vi "1TableGenerateHeaders.vi"(7 "HeaderPrefix":string, 8 "error in (no error)":errorcluster, 11 "Cluster Variant":variant) -> (0 "error out":errorcluster, 1 "LV Data Types":T1[](array[typedef]) format="%.0x", 2 "Headers":string[](array[string]), 3 "Table Name":string)   [LabVIEW 2014, in "TableLogger_Actor.lvlib" / "TableLogger_Actor.lvclass"]
uses:
  TableLogger_Actor.lvclass
  <userlib>/_OpenG.lib/lvdata/lvdata.llb/Type Descriptor Enumeration__ogtk.ctl
panel:
  # "Connector Pane"
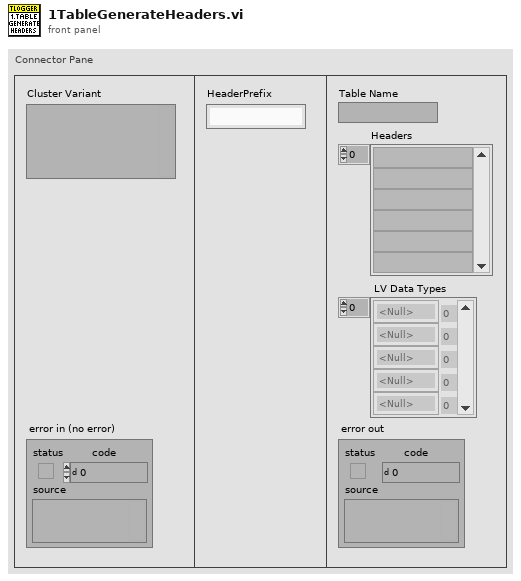
[diagram p1: front panel]
types:
  T1 = typedef "Type Descriptor Enumeration__ogtk.ctl" = enum8{"<Null>", "I8", "I16", "I32", "I64", "U8", "U16", "U32", "U64", "SGL", "DBL", "EXT", "CSG", "CDB", "CXT", "0x0F", "0x10", "0x11", "0x12", "0x13", "0x14", "Enum U8", "Enum U16", "Enum U32", "Enum U64", "SGL PQ", "DBL PQ", "EXT PQ", "CSG PQ", "CDB PQ", "CXT PQ", "0x1F", "0x20", "Boolean", "0x22", "0x23", "0x24", "0x25", "0x26", "0x27", "0x28", "0x29", "0x2A", "0x2B", "0x2C", "0x2D", "0x2E", "0x2F", "String", "0x31", "Path", "Pict", "0x34", "0x35", "0x36", "DAQ", "0x38", "0x39", "0x3A", "0x3B", "0x3C", "0x3D", "0x3E", "0x3F", "Array", "0x41", "0x42", "0x43", "0x44", "0x45", "0x46", "0x47", "0x48", "0x49", "0x4A", "0x4B", "0x4C", "0x4D", "0x4E", "0x4F", "Cluster", "0x51", "0x52", "Variant", "Waveform", "0x55", "0x56", "0x57", "0x58", "0x59", "0x5A", "0x5B", "0x5C", "0x5D", "0x5E", "0x5F", "0x60", "0x61", "0x62", "0x63", "0x64", "0x65", "0x66", "0x67", "0x68", "0x69", "0x6A", "0x6B", "0x6C", "0x6D", "0x6E", "0x6F", "Refnum"}
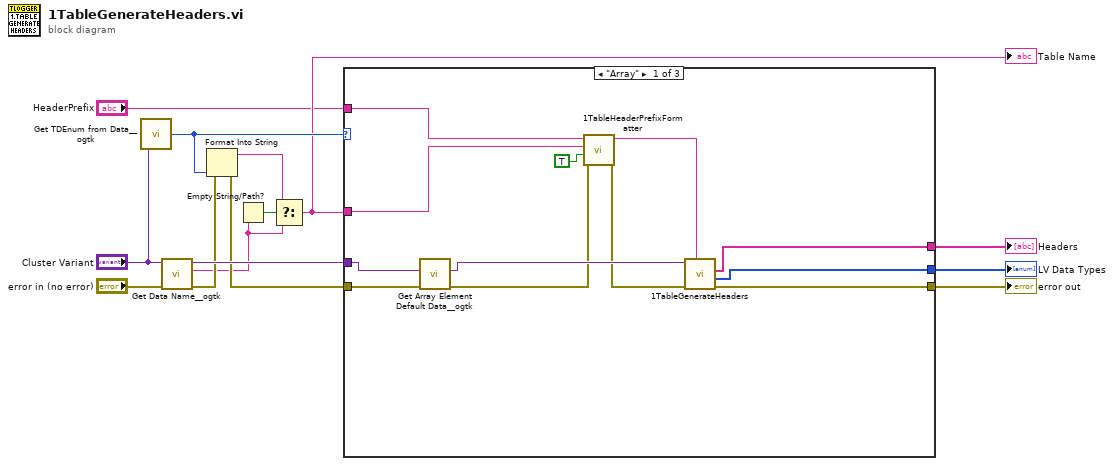
[diagram p0: block diagram]
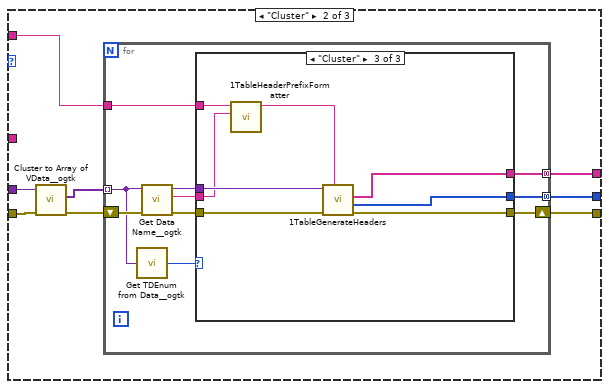
[diagram p2: hidden frame]
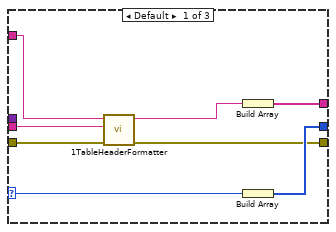
[diagram p3: hidden frame]
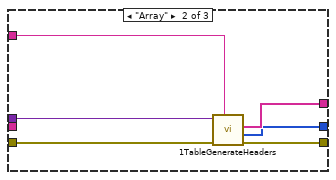
[diagram p4: hidden frame]
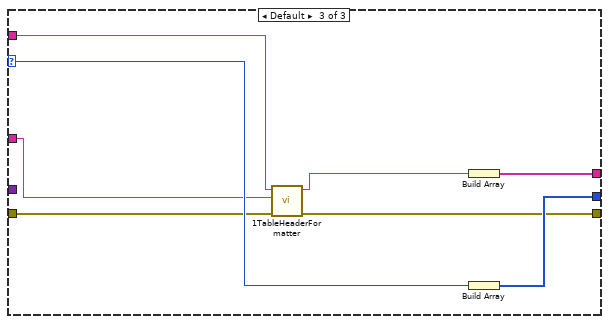
[diagram p5: hidden frame]
diagram:
  n1 = call <userlib>:"Get TDEnum from Data__ogtk.vi"("Data"="Cluster Variant") -> ("Type Descriptor Enumeration"=w7:T1)  [unwired: 4 in]
  n2 = call <userlib>:"Get Data Name__ogtk.vi"("error in (no error)"="error in (no error)", "Data"="Cluster Variant") -> ("error out"=w5:errorcluster, "Data Name"=w3:string, "Data dup"=w9:variant)  [unwired: 7 in]
  n3 = Format Into String(error in=w5, w7) -> (resulting string=w6:string, error out=w4:errorcluster)  [unwired: 2 in]
  n4 = Empty String/Path?(string/path=w3) -> (empty?=w8:bool)
  n5 = Select(t=w6, s=w8, f=w3) -> (s? t:f=w2:string)
  "Table Name" <- w2
  n6 = case shown="\"Array\"" w7 {
    selector: w7 -> [_ _ w72]
    tunnel: w9 -> [w22 w33 _]
    tunnel: [w26 w34 w74] -> w14
    tunnel: w4 -> [w23 w28 w71]
    tunnel: [w25 w30 w70] -> w13
    tunnel: [w21 w29 w73] -> w12
    tunnel: "HeaderPrefix" -> [w20 w27 w69]
    tunnel: w2 -> [w19 _ w68]
    frame "Array" {
      n7 = call <userlib>:"Get Array Element Default Data__ogtk.vi"("error in (no error)"=w23, "Array"=w22) -> ("error out"=w16:errorcluster, "Array Element Default Data"=w24:variant)  [unwired: 8 in]
      n8 = call "1TableHeaderPrefixFormatter.vi"("error in"=w16, "Array?"=TRUE, "Added HeaderPrefix"=w19, "Existing HeaderPrefix"=w20) -> ("error out"=w15:errorcluster, "HeaderPrefix"=w18:string)  [unwired: 6 in]
      n9 = call "1TableGenerateHeaders.vi"("HeaderPrefix"=w18, "error in (no error)"=w15, "Cluster Variant"=w24) -> ("error out"=w25:errorcluster, "LV Data Types"=w21:T1[], "Headers"=w26:string[])  [unwired: 5 in, 1 out]
    }
    frame "Cluster" {
      n10 = call <userlib>:"Cluster to Array of VData__ogtk.vi"("error in (no error)"=w28, "Cluster"=w33) -> ("error out"=w31:errorcluster, "Array of VData"=w32:variant[])  [unwired: 8 in]
      n11 = for {
        tunnel: w32 -> [w38] mode=indexing
        tunnel: [w44] -> w34 mode=concatenating
        shift-right: [w43] -> w30
        shift-left: w31 -> [w40]
        tunnel: [w41] -> w29 mode=concatenating
        tunnel: w27 -> [w35]
        n12 = call <userlib>:"Get TDEnum from Data__ogtk.vi"("Data"=w38) -> ("Type Descriptor Enumeration"=w42:T1)  [unwired: 4 in]
        n13 = call <userlib>:"Get Data Name__ogtk.vi"("error in (no error)"=w40, "Data"=w38) -> ("error out"=w39:errorcluster, "Data Name"=w36:string, "Data dup"=w37:variant)  [unwired: 7 in]
        n14 = case shown="\"Cluster\"" w42 {
          selector: w42 -> [w50 _ _]
          tunnel: w37 -> [_ w57 w66]
          tunnel: [w52 w58 w63] -> w44
          tunnel: w39 -> [w49 w56 w65]
          tunnel: [w48 w55 w64] -> w43
          tunnel: [w51 w54 w62] -> w41
          tunnel: w36 -> [w46 _ w60]
          tunnel: w35 -> [w47 w53 w61]
          frame Default {
            n15 = call "1TableHeaderFormatter.vi"("error in (no error)"=w49, "Data Name"=w46, "HeaderPrefix"=w47) -> ("error out"=w48:errorcluster, "HeaderOut"=w45:string)  [unwired: 7 in]
            n16 = Build Array(w45) -> (w52:string[])
            n17 = Build Array(w50) -> (w51:T1[])
          }
          frame "Array" {
            n18 = call "1TableGenerateHeaders.vi"("HeaderPrefix"=w53, "error in (no error)"=w56, "Cluster Variant"=w57) -> ("error out"=w55:errorcluster, "LV Data Types"=w54:T1[], "Headers"=w58:string[])  [unwired: 5 in, 1 out]
          }
          frame "Cluster" {
            n19 = call "1TableHeaderPrefixFormatter.vi"("Added HeaderPrefix"=w60, "Existing HeaderPrefix"=w61) -> ("HeaderPrefix"=w59:string)  [unwired: 8 in, 1 out]
            n20 = call "1TableGenerateHeaders.vi"("HeaderPrefix"=w59, "error in (no error)"=w65, "Cluster Variant"=w66) -> ("error out"=w64:errorcluster, "LV Data Types"=w62:T1[], "Headers"=w63:string[])  [unwired: 5 in, 1 out]
          }
        }
      }
    }
    frame Default {
      n21 = call "1TableHeaderFormatter.vi"("error in (no error)"=w71, "Data Name"=w68, "HeaderPrefix"=w69) -> ("error out"=w70:errorcluster, "HeaderOut"=w67:string)  [unwired: 7 in]
      n22 = Build Array(w67) -> (w74:string[])
      n23 = Build Array(w72) -> (w73:T1[])
    }
  }
  "Headers" <- w14
  "error out" <- w13
  "LV Data Types" <- w12
